vi "SERIAL_CapturePacket.vi"(11 "Stream":string) -> (0 "Packet Located":bool, 1 "Packet Length":i32, 2 "Packet":string, 3 "Stream":string)   [LabVIEW 2014, in "navX-MXP IMU.lvlib"]
uses:
  navX-MXP IMU.lvlib
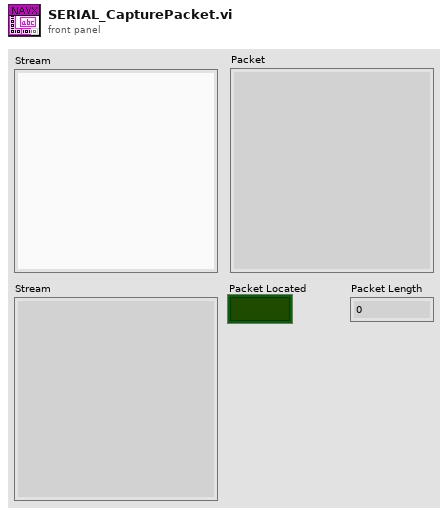
[diagram p1: front panel]
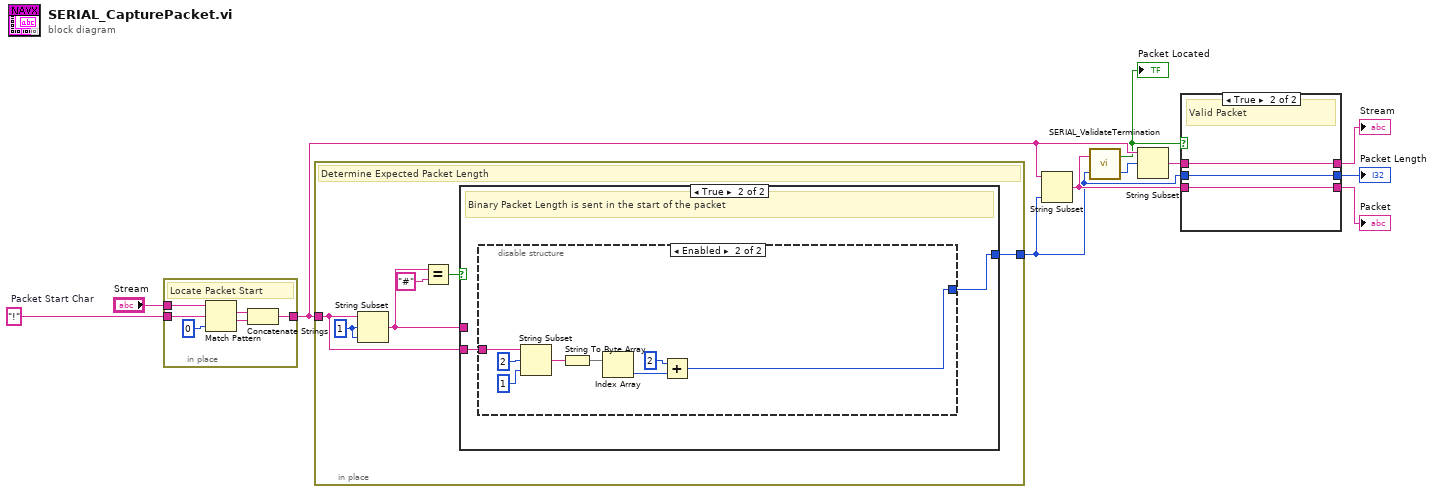
[diagram p0: block diagram]
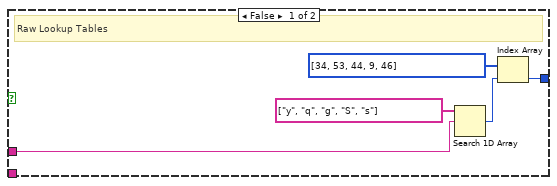
[diagram p2: hidden frame]
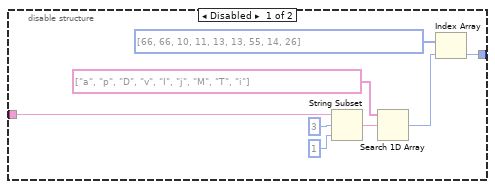
[diagram p3: hidden frame]
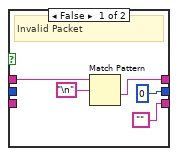
[diagram p4: hidden frame]
diagram:
  w10 = "!"  # Packet Start Char
  n1 = in-place {
    in-place-border: "Stream" -> [w16]
    in-place-border: [w13] -> w5
    in-place-border: w10 -> [w12]
    # "Locate Packet Start"
    n2 = Match Pattern(string=w16, regular expression=w12, offset (0)=0 ("offset past match")) -> (match substring=w15:string, after substring=w14:string)  [unwired: 2 out]
    n3 = Concatenate Strings(w15, w14) -> (w13:string)
  }
  n4 = in-place {
    in-place-border: w5 -> [w19]
    in-place-border: [w18] -> w1
    w23 = 1 ("length (rest)")
    # "Determine Expected Packet Length"
    n5 = String Subset(string=w19, offset (0)=w23, length (rest)=w23) -> (substring=w20:string)
    n6 = Equal?(x=w20, y="#" ("Binay Packet Indicator Char")) -> (x = y?=w21:bool)
    n7 = case shown="True" w21 {
      tunnel: w20 -> [w27 _]
      tunnel: [w24 w30] -> w18
      tunnel: w19 -> [_ w29]
      frame False {
        # "Raw Lookup Tables"
        n8 = Search 1D Array(1D array=string[] ["y", "q", "g", "S", "s"], element=w27) -> (index of element=w25:i32)  [unwired: 1 in]
        n9 = Index Array(array=i32[] [34, 53, 44, 9, 46], index=w25) -> (element=w24:i32)
      }
      frame True {
        # "Binary Packet Length is sent in the start of the packet"
        n10 = disable-structure shown="Enabled" {
          disable-tunnel: [w32 w39] -> w30
          disable-tunnel: w29 -> [w31 w40]
          frame Disabled {
            n11 = String Subset(string=w31, offset (0)=3, length (rest)=1 ("length (rest)")) -> (substring=w33:string)
            n12 = Search 1D Array(1D array=string[] ["a", "p", "D", "v", "I", "j", "M", "T", "i"], element=w33) -> (index of element=w38:i32)  [unwired: 1 in]
            n13 = Index Array(array=i32[] [66, 66, 10, 11, 13, 13, 55, 14, 26], index=w38) -> (element=w32:i32)
          }
          frame Enabled {
            n14 = String Subset(string=w40, offset (0)=2, length (rest)=1 ("length (rest)")) -> (substring=w43:string)
            n15 = String To Byte Array(string=w43) -> (unsigned byte array=w44:u8[])
            n16 = Index Array(array=w44) -> (element=w45:u8)  [unwired: 1 in]
            n17 = Add(x=u8 2 ("y"), y=w45) -> (x+y=w39:u8)
          }
        }
      }
    }
  }
  n18 = String Subset(string=w5, length (rest)=w1) -> (substring=w2:string)  [unwired: 1 in]
  n19 = call "SERIAL_ValidateTermination.vi"("Expected Packet Length"=w1, "Content"=w2) -> ("Termination Offset"=w3:i32, "Valid?"=w4:bool)
  "Packet Located" <- w4
  n20 = String Subset(string=w5, offset (0)=w3) -> (substring=w6:string)  [unwired: 1 in]
  n21 = case shown="True" w4 {
    tunnel: w6 -> [w51 w54]
    tunnel: [w50 w54] -> w8
    tunnel: w1 -> [_ w53]
    tunnel: [0 ("Packet Length") w53] -> w7
    tunnel: ["" w52] -> w9
    tunnel: w2 -> [_ w52]
    frame False {
      # "Invalid Packet"
      n22 = Match Pattern(string=w51, regular expression="\n") -> (after substring=w50:string)  [unwired: 1 in, 3 out]
    }
    frame True {
      # "Valid Packet"
    }
  }
  "Packet" <- w9
  "Stream" <- w8
  "Packet Length" <- w7
